vi "Begin.vi"(8 "error in":errorcluster) -> (0 "error out":errorcluster)   [LabVIEW 2017]
doc: "Called before other user functions, this VI can be used to open I/O refnums, load in file data, and do general program initialization. Notice that the <B>error out</B> terminal is simply used for data flow. Wiring it to other structures or subVIs ensures that this VI runs first."
uses:
  <vilib>/Rock Robotics/SystemInterfaces/spilib/spi_bus.ctl
  VIs/CtrlRefs/SettingsALB.ctl
  <vilib>/Rock Robotics/WPI/DriverStation/WPI_DriverStationRobotMode2.ctl
  <vilib>/Rock Robotics/WPI/Joystick/WPI_JoystickDeviceEnum.ctl
  <vilib>/Rock Robotics/SystemInterfaces/DIO/FPGA_DIOPWMChannel.ctl
  <vilib>/Rock Robotics/WPI/SafetyOutput/WPI_SafetyOutputConfigMenu.ctl
  <vilib>/Rock Robotics/SystemInterfaces/DIO/FPGA_DIOChannel.ctl
  <vilib>/Rock Robotics/Network Tables/NT Write Boolean.vi
  <vilib>/Rock Robotics/Network Tables/NT Write String Array.vi
  Robot Global Data.vi
  <vilib>/Rock Robotics/WPI/RobotDrive/WPI_RobotDriveOpen4MotorWithTalonSRX.vi
  <vilib>/Rock Robotics/WPI/Gyro/WPI_GyroXRS450_SPI_Open.vi
  <vilib>/Rock Robotics/WPI/MotorControl/WPI_MotorControlOpen VictorSP.vi
  <vilib>/Rock Robotics/WPI/Switch/WPI_SwitchOpenLimit.vi
  <vilib>/Rock Robotics/SystemInterfaces/DIO/FPGA_DIORelayChannel.ctl
panel:
  out "Device Found":bool
  in  "SPI Bus":T1
  in  "Sample Rate (Hz)":dbl=1000.0 min=50.0 max=20000.0 format="%#_13g"
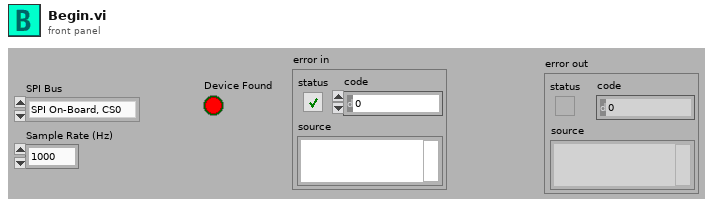
[diagram p1: front panel]
types:
  T1 = typedef "spi_bus.ctl" = enum16{"SPI On-Board, CS0", "SPI On-Board, CS1", "SPI On-Board, CS2", "SPI On-Board, CS3", "SPI MXP", "Invalid"}
  T2 = typedef "WPI_JoystickDeviceEnum.ctl" = enum16{"USB 0", "USB 1", "USB 2", "USB 3", "USB 4", "USB 5"}
  T3 = typedef "WPI_DriverStationRobotMode2.ctl" = enum16{"Autonomous Disabled", "Autonomous Enabled", "Teleop Disabled", "Teleop Enabled", "Disconnected", "Finish", "Test Disabled", "Test Enabled", "Emergency Stopped"}
  T4 = typedef "FPGA_DIORelayChannel.ctl" = enum8{"Relay 0", "Relay 1", "Relay 2", "Relay 3", "Invalid"}
  T5 = typedef "WPI_SafetyOutputConfigMenu.ctl" = enum16{"Enable", "Disable"}
  T6 = typedef "FPGA_DIOPWMChannel.ctl" = enum8{"PWM 0", "PWM 1", "PWM 2", "PWM 3", "PWM 4", "PWM 5", "PWM 6", "PWM 7", "PWM 8", "PWM 9", "PWM MXP 0", "PWM MXP 1", "PWM MXP 2", "PWM MXP 3", "PWM MXP 4", "PWM MXP 5", "PWM MXP 6", "PWM MXP 7", "PWM MXP 8", "PWM MXP 9", "Invalid"}
  T7 = typedef "FPGA_DIOChannel.ctl" = enum8{"DIO 0", "DIO 1", "DIO 2", "DIO 3", "DIO 4", "DIO 5", "DIO 6", "DIO 7", "DIO 8", "DIO 9", "DIO MXP 0", "DIO MXP 1", "DIO MXP 2", "DIO MXP 3", "DIO MXP 4", "DIO MXP 5", "DIO MXP 6", "DIO MXP 7", "DIO MXP 8", "DIO MXP 9", "DIO MXP 10", "DIO MXP 11", "DIO MXP 12", "DIO MXP 13", "DIO MXP 14", "DIO MXP 15", "SPI Port CS1", "SPI Port CS2", "SPI Port CS3", "SPI Port MISO", "SPI Port MOSI", "Invalid"}
  T8 = typedef "MacrosALB.ctl" = cluster{"MacroName":string, "Sequence":cluster{"Buttons 1":T9, "Axes 1":T10, "Buttons 2":T11, "Axes 2":T12, "Delay":u32}[], "TotalTime":u32}
  T9 = typedef "JoyStick1ALB.ctl" = cluster{"J1-B0":bool, "J1-B1":bool, "J1-B2":bool, "J1-B3":bool, "J1-B4":bool, "J1-B5":bool, "J1-B6":bool, "J1-B7":bool, "J1-B8-":bool, "J1-B9":bool, "J1-B10":bool, "J1-B11":bool}
  T10 = typedef "JoyStick1ALV(Analog).ctl" = cluster{"Axis 0":dbl, "Axis 1":dbl, "Axis 2":dbl, "Slider":dbl}
  T11 = typedef "JoyStick2ALB.ctl" = cluster{"J2-B0":bool, "J2-B1":bool, "J2-B2":bool, "J2-B3":bool, "J2-B4":bool, "J2-B5":bool, "J2-B6":bool, "J2-B7":bool, "J2-B8":bool, "J2-B9":bool, "J2-B10":bool, "J2-B11":bool}
  T12 = typedef "JoyStick2ALB(Analog).ctl" = cluster{"Axis 0":dbl, "Axis 1":dbl, "Axis 2":dbl, "Switch":dbl}
  T13 = typedef "SettingsALB.ctl" = cluster{"Unused 1":dbl, "Unused 2":dbl, "Unused 3":dbl, "Unused 4":dbl, "Unused 5":dbl, "Unused 6":dbl, "Unused 7":dbl, "Unused 8":dbl, "Unused 9":dbl, "Unused 10":dbl, "Unused 11":dbl, "Unused 12":dbl}
  T14 = typedef "WPI_JoystickDevRef.ctl" = cluster{"Device":T2}
  T15 = typedef "WPI_RelayDevRef.ctl" = cluster{"DevStatus":errorcluster, "Relay Channel":T4, "Relay Direction":T16}
  T16 = typedef "WPI_RelayDirection.ctl" = enum16{"Both directions", "Forward only", "Reverse only"}
  T17 = typedef "WPI_GyroDevRef.ctl" = cluster{"DevStatus":errorcluster, "Analog Channel":T18, "Gain (VoltsPerDegree/Second)":dbl, "Gyro Type":enum16{"Analog", "XRS450"}, "Handle":i32, "SPI Bus":T1, "Device Found":bool, "Sample Rate":dbl, "Calibrate On Open":bool, "Offset":dbl}
  T18 = typedef "FPGA_AIChannel.ctl" = enum8{"AI 0", "AI 1", "AI 2", "AI 3", "AI MXP 0", "AI MXP 1", "AI MXP 2", "AI MXP 3", "Invalid"}
  T19 = typedef "WPI_RobotDriveDevRef.ctl" = cluster{"DevStatus":errorcluster, "Motors[]":T20[], "Square Inputs":bool, "Max Output":dbl}
  T20 = typedef "WPI_MotorControlDeviceRef.ctl" = cluster{"DeviceStatus":errorcluster, "Type":T21, "PWM":cluster{"PWM Channel":T6, "DeadBand":T22}, "CAN":cluster{"Device Number":u8, "SetOutput VI Ref":variant, "GetOutput VI Ref":variant, "Enable VI Ref":variant, "Disable VI Ref":variant, "Data":variant}, "Invert":bool, "DIO PWM":cluster{"PWM \"Enable\" Channel":T6, "DIOChannel":T7, "PWM Rate":dbl}}
  T21 = typedef "WPI_MotorControlType.ctl" = enum16{"PWM", "CAN", "DIO PWM"}
  T22 = typedef "WPI_PWMDeadband.ctl" = cluster{"Name":string, "maxPositivePwm":i32, "minPositivePwm":i32, "centerPwm":i32, "maxNegativePwm":i32, "minNegativePwm":i32, "angularRange":u16}
  T23 = typedef "WPI_SwitchDevRef.ctl" = cluster{"DevStatus":errorcluster, "DIO Channel":T7, "CntIndex":T24, "Normally Closed":bool}
  T24 = typedef "FPGA_CounterCtrSystemIndex.ctl" = enum8{"Ctr 0", "Ctr 1", "Ctr 2", "Ctr 3", "Ctr 4", "Ctr 5", "Ctr 6", "Ctr 7", "Invalid"}
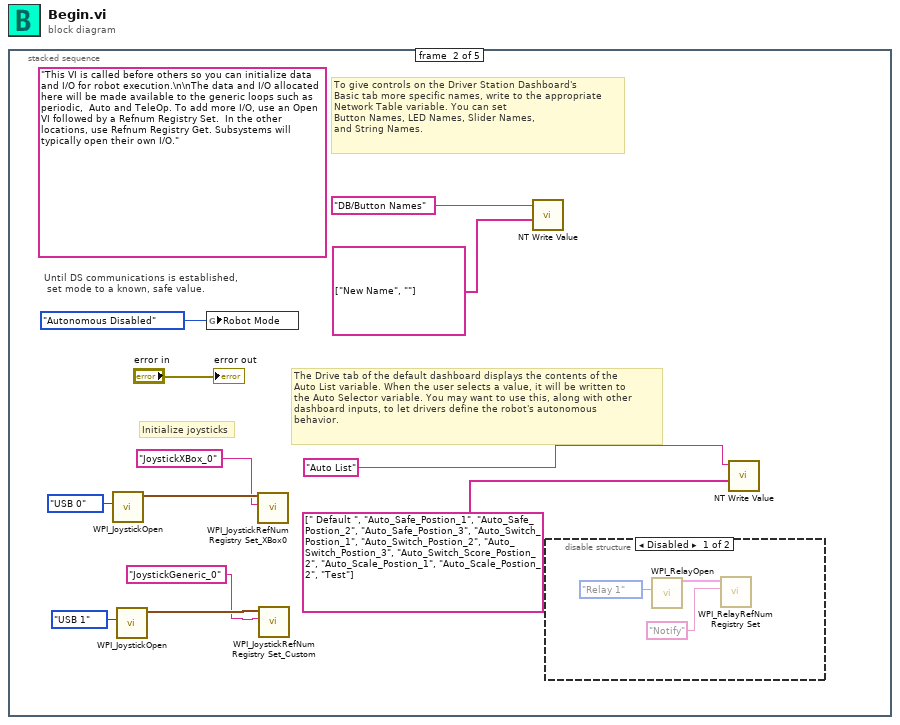
[diagram p0: block diagram]
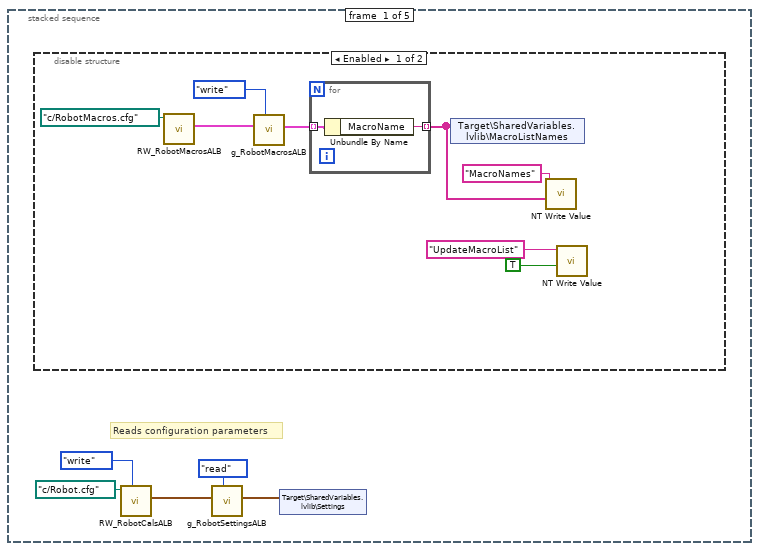
[diagram p2: hidden frame]
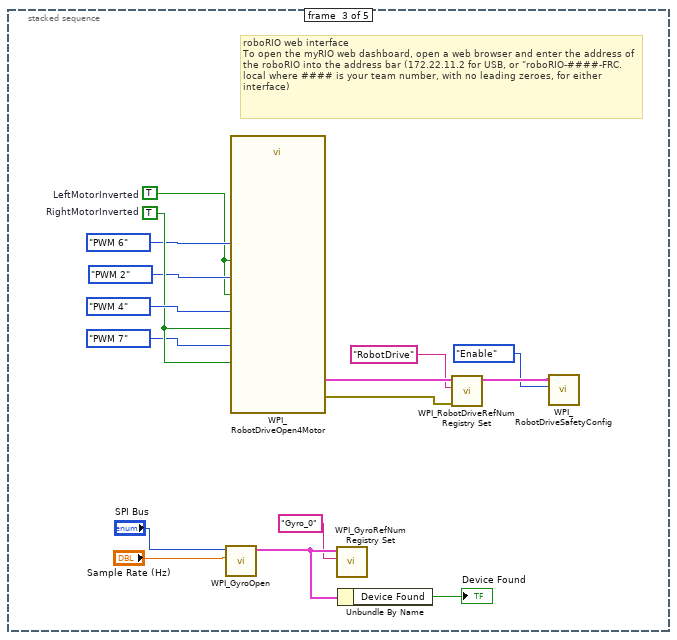
[diagram p5: hidden frame]
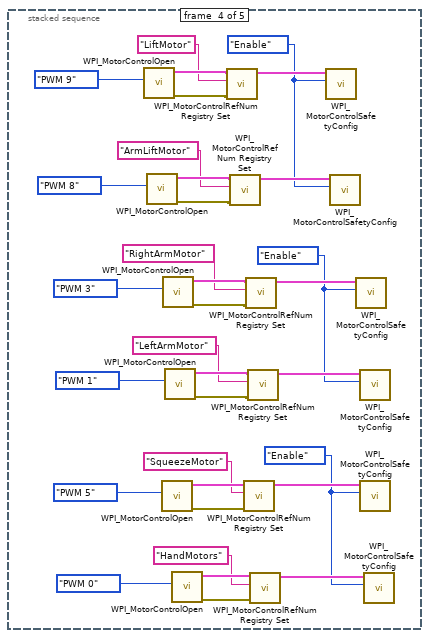
[diagram p6: hidden frame]
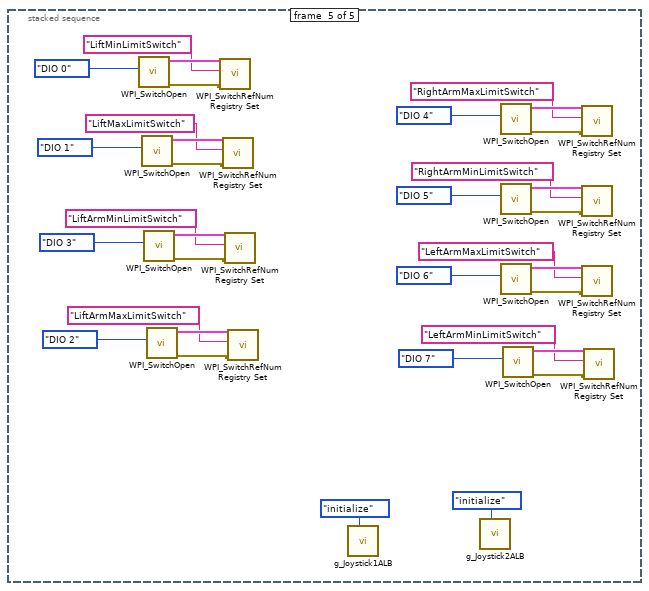
[diagram p7: hidden frame]
diagram:
  n1 = stacked-sequence {
    frame #0 {
      # "Reads configuration parameters"
      n2 = disable-structure shown="Enabled" {
        frame Enabled {
          n3 = call "RW_RobotMacrosALB.vi"("File Path"=path "c:/RobotMacros.cfg") -> ("Macros out"=w13:T8[])  [unwired: 9 in, 1 out]
          n4 = call "g_RobotMacrosALB.vi"("Action"=enum16{"read", "write"}."write", "Macros"=w13) -> ("Macros out"=w11:T8[])  [unwired: 9 in]
          n5 = for {
            tunnel: w11 -> [w15] mode=indexing
            tunnel: [w14] -> w9 mode=indexing
            n6 = Unbundle By Name(w15) -> ("MacroName"=w14:string)
          }
          n7 = shared-variable "Target\\SharedVariables.lvlib\\MacroListNames"(w9) -> ()  [unwired: 1 in, 1 out]
          n8 = call-poly <vilib>:"NT Write Value.vi"("String Array"=w9, "Name"="MacroNames") -> ()  [unwired: 9 in, 1 out]
          n9 = call-poly <vilib>:"NT Write Value.vi"("Boolean"=TRUE, "Name"="UpdateMacroList") -> ()  [unwired: 9 in, 1 out]
        }
        frame Disabled {
        }
      }
      n10 = call "RW_RobotCalsALB.vi"("Action"=enum16{"read", "write"}."write", "File Path"=path "c:/Robot.cfg") -> ("Settings out"=w2:T13)  [unwired: 8 in, 1 out]
      n11 = call "g_RobotSettingsALB.vi"("Action"=enum16{"read", "write"}."read", "Settings"=w2) -> ("Settings out"=w1:T13)  [unwired: 9 in]
      n12 = shared-variable "Target\\SharedVariables.lvlib\\Settings"(w1) -> ()  [unwired: 1 in, 1 out]
    }
    frame #1 {
      (unwired) "This VI is called before others so you can initialize data and I/O for robot execution.\n\nThe data and I/O allocated here will be made available to the generic loops such as periodic,  Auto and TeleOp. To add more I/O, use an Open VI followed by a Refnum Registry Set.  In the other locations, use Refnum Registry Get. Subsystems will typically open their own I/O."
      # "The Drive tab of the default dashboard displays the contents of the\nAuto List variable. When the user selects a value, it will be written to\nthe Auto Selector variable. You may want to use this, along with other\ndashboard inputs, to let drivers define the robot's autonomous\nbehavior."
      # "To give controls on the Driver Station Dashboard's\nBasic tab more specific names, write to the appropriate\nNetwork Table variable. You can set\nButton Names, LED Names, Slider Names,\nand String Names."
      # "Initialize joysticks"
      # "Until DS communications is established,\n set mode to a known, safe value."
      n13 = call <vilib>:"WPI_JoystickOpen.vi"("JoystickDevice"=WPI_JoystickDeviceEnum."USB 0") -> ("JoystickDevRef"=w20:T14)  [unwired: 10 in]
      n14 = call <vilib>:"WPI_JoystickOpen.vi"("JoystickDevice"=WPI_JoystickDeviceEnum."USB 1") -> ("JoystickDevRef"=w18:T14)  [unwired: 10 in]
      n15 = global write "Robot Global Data.vi" "Robot Mode"(WPI_DriverStationRobotMode2."Autonomous Disabled" ("Robot Mode")) -> ()
      n16 = call "WPI_JoystickRefNum Registry Set_XBox0.vi"("refnum name"="JoystickXBox_0", "DevRef"=w20) -> ()  [unwired: 8 in, 2 out]
      n17 = call "WPI_JoystickRefNum Registry Set_Custom.vi"("refnum name"="JoystickGeneric_0", "DevRef"=w18) -> ()  [unwired: 8 in, 2 out]
      n18 = call-poly <vilib>:"NT Write Value.vi"("String Array"=string[] ["New Name", ""], "Name"="DB/Button Names") -> ()  [unwired: 9 in, 1 out]
      n19 = disable-structure shown="Disabled" {
        frame Disabled {
          n20 = call <vilib>:"WPI_RelayOpen.vi"("Relay Channel"=FPGA_DIORelayChannel."Relay 1") -> ("RelayDevRef"=w29:T15)  [unwired: 9 in, 1 out]
          n21 = call <vilib>:"WPI_RelayRefNum Registry Set.vi"("refnum name"="Notify", "RelayDevRef"=w29) -> ()  [unwired: 8 in, 2 out]
        }
        frame Enabled {
        }
      }
      n22 = call-poly <vilib>:"NT Write Value.vi"("String Array"=string[] [" Default ", "Auto_Safe_Postion_1", "Auto_Safe_Postion_2", "Auto_Safe_Postion_3", "Auto_Switch_Postion_1", "Auto_Switch_Postion_2", "Auto_Switch_Postion_3", "Auto_Switch_Score_Postion_2", "Auto_Scale_Postion_1", "Auto_Scale_Postion_2", "Test"], "Name"="Auto List") -> ()  [unwired: 9 in, 1 out]
      "error out" <- "error in"
    }
    frame #2 {
      w36 = TRUE  # LeftMotorInverted
      w40 = TRUE  # RightMotorInverted
      # "roboRIO web interface\nTo open the myRIO web dashboard, open a web browser and enter the address of the roboRIO into the address bar (172.22.11.2 for USB, or \"roboRIO-####-FRC.local where #### is your team number, with no leading zeroes, for either interface)"
      n23 = call-poly <vilib>:"WPI_GyroOpen.vi"("Sample Rate (Hz)"="Sample Rate (Hz)", "SPI Bus"="SPI Bus") -> ("GyroDevRef"=w34:T17)  [unwired: 7 in, 2 out]
      n24 = call-poly <vilib>:"WPI_RobotDriveOpen4Motor.vi"("Rear Left Motor"=FPGA_DIOPWMChannel."PWM 4", "Rear Left Motor Inverted"=w40, "Rear Right Motor Inverted"=w40, "Rear Right Motor"=FPGA_DIOPWMChannel."PWM 7", "Front Left Motor"=FPGA_DIOPWMChannel."PWM 6" ("Rear Left Motor"), "Front Right Motor"=FPGA_DIOPWMChannel."PWM 2", "Front Left Motor Inverted"=w36, "Front Right Motor Inverted"=w36) -> ("RobotDriveDevRef"=w45:T19, "error out"=w44:errorcluster)  [unwired: 6 in]
      n25 = call <vilib>:"WPI_GyroRefNum Registry Set.vi"("refnum name"="Gyro_0", "GyroDevRef"=w34) -> ()  [unwired: 8 in, 2 out]
      n26 = Unbundle By Name(w34) -> ("Device Found"=→"Device Found":bool)
      n27 = call <vilib>:"WPI_RobotDriveRefNum Registry Set.vi"("error in (no error)"=w44, "refnum name"="RobotDrive", "RobotDriveDevRef"=w45) -> ("RobotDriveDevRef"=w46:T19)  [unwired: 7 in, 1 out]
      n28 = call <vilib>:"WPI_RobotDriveSafetyConfig.vi"("mode"=WPI_SafetyOutputConfigMenu."Enable", "RobotDriveDevRef"=w46) -> ()  [unwired: 8 in, 2 out]
    }
    frame #3 {
      w51 = WPI_SafetyOutputConfigMenu."Enable" ("mode")
      w62 = WPI_SafetyOutputConfigMenu."Enable" ("mode")
      w73 = WPI_SafetyOutputConfigMenu."Enable" ("mode")
      n29 = call-poly <vilib>:"WPI_MotorControlOpen.vi"("PWM Channel"=FPGA_DIOPWMChannel."PWM 9") -> ("error out"=w75:errorcluster, "MotorControlDeviceRef"=w74:T20)  [unwired: 9 in]
      n30 = call-poly <vilib>:"WPI_MotorControlOpen.vi"("PWM Channel"=FPGA_DIOPWMChannel."PWM 8") -> ("error out"=w77:errorcluster, "MotorControlDeviceRef"=w76:T20)  [unwired: 9 in]
      n31 = call-poly <vilib>:"WPI_MotorControlOpen.vi"("PWM Channel"=FPGA_DIOPWMChannel."PWM 5") -> ("error out"=w55:errorcluster, "MotorControlDeviceRef"=w54:T20)  [unwired: 9 in]
      n32 = call-poly <vilib>:"WPI_MotorControlOpen.vi"("PWM Channel"=FPGA_DIOPWMChannel."PWM 3") -> ("error out"=w64:errorcluster, "MotorControlDeviceRef"=w63:T20)  [unwired: 9 in]
      n33 = call-poly <vilib>:"WPI_MotorControlOpen.vi"("PWM Channel"=FPGA_DIOPWMChannel."PWM 1") -> ("error out"=w66:errorcluster, "MotorControlDeviceRef"=w65:T20)  [unwired: 9 in]
      n34 = call-poly <vilib>:"WPI_MotorControlOpen.vi"("PWM Channel"=FPGA_DIOPWMChannel."PWM 0") -> ("error out"=w52:errorcluster, "MotorControlDeviceRef"=w53:T20)  [unwired: 9 in]
      n35 = call <vilib>:"WPI_MotorControlRefNum Registry Set.vi"("error in (no error)"=w75, "refnum name"="LiftMotor", "MotorControlDevRef"=w74) -> ("MotorControlDevRef"=w78:T20)  [unwired: 7 in, 1 out]
      n36 = call <vilib>:"WPI_MotorControlRefNum Registry Set.vi"("error in (no error)"=w77, "refnum name"="ArmLiftMotor", "MotorControlDevRef"=w76) -> ("MotorControlDevRef"=w79:T20)  [unwired: 7 in, 1 out]
      n37 = call <vilib>:"WPI_MotorControlRefNum Registry Set.vi"("error in (no error)"=w55, "refnum name"="SqueezeMotor", "MotorControlDevRef"=w54) -> ("MotorControlDevRef"=w56:T20)  [unwired: 7 in, 1 out]
      n38 = call <vilib>:"WPI_MotorControlRefNum Registry Set.vi"("error in (no error)"=w64, "refnum name"="RightArmMotor", "MotorControlDevRef"=w63) -> ("MotorControlDevRef"=w67:T20)  [unwired: 7 in, 1 out]
      n39 = call <vilib>:"WPI_MotorControlRefNum Registry Set.vi"("error in (no error)"=w66, "refnum name"="LeftArmMotor", "MotorControlDevRef"=w65) -> ("MotorControlDevRef"=w68:T20)  [unwired: 7 in, 1 out]
      n40 = call <vilib>:"WPI_MotorControlRefNum Registry Set.vi"("error in (no error)"=w52, "refnum name"="HandMotors", "MotorControlDevRef"=w53) -> ("MotorControlDevRef"=w57:T20)  [unwired: 7 in, 1 out]
      n41 = call <vilib>:"WPI_MotorControlSafetyConfig.vi"("mode"=w73, "MotorControlDevRef"=w78) -> ()  [unwired: 8 in, 2 out]
      n42 = call <vilib>:"WPI_MotorControlSafetyConfig.vi"("mode"=w73, "MotorControlDevRef"=w79) -> ()  [unwired: 8 in, 2 out]
      n43 = call <vilib>:"WPI_MotorControlSafetyConfig.vi"("mode"=w62, "MotorControlDevRef"=w67) -> ()  [unwired: 8 in, 2 out]
      n44 = call <vilib>:"WPI_MotorControlSafetyConfig.vi"("mode"=w62, "MotorControlDevRef"=w68) -> ()  [unwired: 8 in, 2 out]
      n45 = call <vilib>:"WPI_MotorControlSafetyConfig.vi"("mode"=w51, "MotorControlDevRef"=w56) -> ()  [unwired: 8 in, 2 out]
      n46 = call <vilib>:"WPI_MotorControlSafetyConfig.vi"("mode"=w51, "MotorControlDevRef"=w57) -> ()  [unwired: 8 in, 2 out]
    }
    frame #4 {
      n47 = call-poly <vilib>:"WPI_SwitchOpen.vi"("DIO Channel"=FPGA_DIOChannel."DIO 0") -> ("error out"=w108:errorcluster, "SwitchDevRef"=w109:T23)  [unwired: 9 in]
      n48 = call-poly <vilib>:"WPI_SwitchOpen.vi"("DIO Channel"=FPGA_DIOChannel."DIO 1") -> ("error out"=w106:errorcluster, "SwitchDevRef"=w107:T23)  [unwired: 9 in]
      n49 = call-poly <vilib>:"WPI_SwitchOpen.vi"("DIO Channel"=FPGA_DIOChannel."DIO 3") -> ("error out"=w112:errorcluster, "SwitchDevRef"=w113:T23)  [unwired: 9 in]
      n50 = call-poly <vilib>:"WPI_SwitchOpen.vi"("DIO Channel"=FPGA_DIOChannel."DIO 2") -> ("error out"=w110:errorcluster, "SwitchDevRef"=w111:T23)  [unwired: 9 in]
      n51 = call <vilib>:"WPI_SwitchRefNum Registry Set.vi"("error in (no error)"=w108, "refnum name"="LiftMinLimitSwitch", "SwitchDevRef"=w109) -> ()  [unwired: 7 in, 2 out]
      n52 = call <vilib>:"WPI_SwitchRefNum Registry Set.vi"("error in (no error)"=w106, "refnum name"="LiftMaxLimitSwitch", "SwitchDevRef"=w107) -> ()  [unwired: 7 in, 2 out]
      n53 = call <vilib>:"WPI_SwitchRefNum Registry Set.vi"("error in (no error)"=w112, "refnum name"="LiftArmMinLimitSwitch", "SwitchDevRef"=w113) -> ()  [unwired: 7 in, 2 out]
      n54 = call <vilib>:"WPI_SwitchRefNum Registry Set.vi"("error in (no error)"=w110, "refnum name"="LiftArmMaxLimitSwitch", "SwitchDevRef"=w111) -> ()  [unwired: 7 in, 2 out]
      n55 = call "g_Joystick1ALB.vi"("Action"=enum16{"initialize", "read", "write"}."initialize") -> ()  [unwired: 7 in, 4 out]
      n56 = call "g_Joystick2ALB.vi"("Action"=enum16{"initialize", "read", "write"}."initialize") -> ()  [unwired: 7 in, 4 out]
      n57 = call-poly <vilib>:"WPI_SwitchOpen.vi"("DIO Channel"=FPGA_DIOChannel."DIO 4") -> ("error out"=w90:errorcluster, "SwitchDevRef"=w91:T23)  [unwired: 9 in]
      n58 = call-poly <vilib>:"WPI_SwitchOpen.vi"("DIO Channel"=FPGA_DIOChannel."DIO 5") -> ("error out"=w92:errorcluster, "SwitchDevRef"=w93:T23)  [unwired: 9 in]
      n59 = call-poly <vilib>:"WPI_SwitchOpen.vi"("DIO Channel"=FPGA_DIOChannel."DIO 6") -> ("error out"=w94:errorcluster, "SwitchDevRef"=w95:T23)  [unwired: 9 in]
      n60 = call-poly <vilib>:"WPI_SwitchOpen.vi"("DIO Channel"=FPGA_DIOChannel."DIO 7") -> ("error out"=w96:errorcluster, "SwitchDevRef"=w97:T23)  [unwired: 9 in]
      n61 = call <vilib>:"WPI_SwitchRefNum Registry Set.vi"("error in (no error)"=w90, "refnum name"="RightArmMaxLimitSwitch", "SwitchDevRef"=w91) -> ()  [unwired: 7 in, 2 out]
      n62 = call <vilib>:"WPI_SwitchRefNum Registry Set.vi"("error in (no error)"=w92, "refnum name"="RightArmMinLimitSwitch", "SwitchDevRef"=w93) -> ()  [unwired: 7 in, 2 out]
      n63 = call <vilib>:"WPI_SwitchRefNum Registry Set.vi"("error in (no error)"=w94, "refnum name"="LeftArmMaxLimitSwitch", "SwitchDevRef"=w95) -> ()  [unwired: 7 in, 2 out]
      n64 = call <vilib>:"WPI_SwitchRefNum Registry Set.vi"("error in (no error)"=w96, "refnum name"="LeftArmMinLimitSwitch", "SwitchDevRef"=w97) -> ()  [unwired: 7 in, 2 out]
    }
  }
